vi "Measurement Logic.vi"() -> ()   [LabVIEW 2021, in "Quiescent Current_Channel Ganging.lvlib"]
uses:
  Quiescent Current_Channel Ganging.lvlib
  <vilib>/Plug-In SDKs/Measurements/Measure Call Context/Measure Call Context.lvclass
  Measurement Configuration.ctl
  Measurement Results.ctl
  <instrlib>/niDCPower/nidcpower.llb/niDCPower Source Mode.ctl
  <instrlib>/niDCPower/nidcpower.llb/niDCPower Output Function.ctl
panel:
  out "measurement results":T1
  in  "measurement configuration":T2={"DUT setup time"=1.0, "Source delay"=0.005, "Aperture time"=0.005, "Source master resource name"="Lorem ipsum dolor sit", "Source slave resource names"=["", ""], "Source system configuration"=enum."Parallel", "Source start voltage"=1.0, "Source stop voltage"=1.0, "Source voltage sweep points"=1, "Source voltage level range"=32.0, "Source sense"=-64, "Source limit symmetry"=enum."Asymmetric", "Source current limit range"=64.0, "Source current limit low"=-32.0, "Source current limit high"=-32.0, "Source transient response"=-64, "Source voltage gain bandwidth"=1.0, "Source voltage compensation frequency"=3530.0, "Source voltage pole-zero ratio"=2.0} {"Source start voltage" format="%#_6p"; "Source sense" items=["Local"=1008, "Remote"=1009]; "Source transient response" items=["Slow"=1041, "Normal"=1038, "Fast"=1039, "Custom"=1042]; "Source voltage level range" format="%#_6p"}
  out "measure call context out":refnum<class "Measure Call Context.lvclass">
  in  "measure call context in":refnum<class "Measure Call Context.lvclass">
  out "error out":errorcluster
  in  "error in":errorcluster
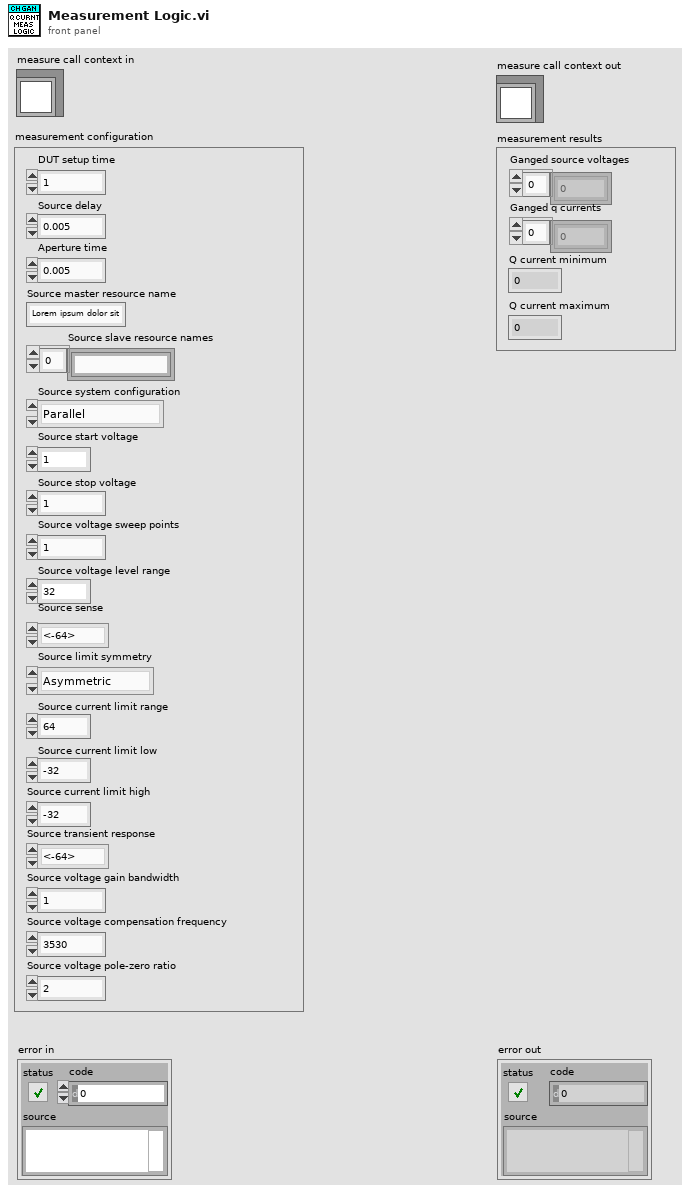
[diagram p1: front panel]
types:
  T1 = typedef "Quiescent Current_Channel Ganging.lvlib/Measurement Results.ctl" = cluster{"Ganged source voltages":dbl[], "Ganged q currents":dbl[], "Q current minimum":dbl, "Q current maximum":dbl}
  T2 = typedef "Quiescent Current_Channel Ganging.lvlib/Measurement Configuration.ctl" = cluster{"DUT setup time":dbl, "Source delay":dbl, "Aperture time":dbl, "Source master resource name":string, "Source slave resource names":string[], "Source system configuration":enum32{"Series", "Parallel", "Manual"}, "Source start voltage":dbl, "Source stop voltage":dbl, "Source voltage sweep points":i32, "Source voltage level range":dbl, "Source sense":i32, "Source limit symmetry":enum32{"Symmetric", "Asymmetric"}, "Source current limit range":dbl, "Source current limit low":dbl, "Source current limit high":dbl, "Source transient response":i32, "Source voltage gain bandwidth":dbl, "Source voltage compensation frequency":dbl, "Source voltage pole-zero ratio":dbl}
  T3 = typedef "niDCPower Output Function.ctl" = i32
  T4 = typedef "niDCPower Source Mode.ctl" = i32
  T5 = typedef "NIDCPower_channel_ganging - ctl - channel def.ctl" = cluster{"resource name":refnum<k15>, "channels":string, "Channel Mode":T6}
  T6 = typedef "NIDCPower_channel_ganging - ctl - channel mode.ctl" = enum32{"Master", "Slave", "Slave - Inverted"}
  T7 = typedef "NIDCPower_channel_ganging - ctl - ganged session.ctl" = cluster{"Ganged Config":T8, "Session List":refnum<k15>[], "Session Mode":T6[], "Channel":string[]}
  T8 = typedef "NIDCPower_channel_ganging - ctl - ganged config.ctl" = enum32{"Series", "Parallel", "Manual"}
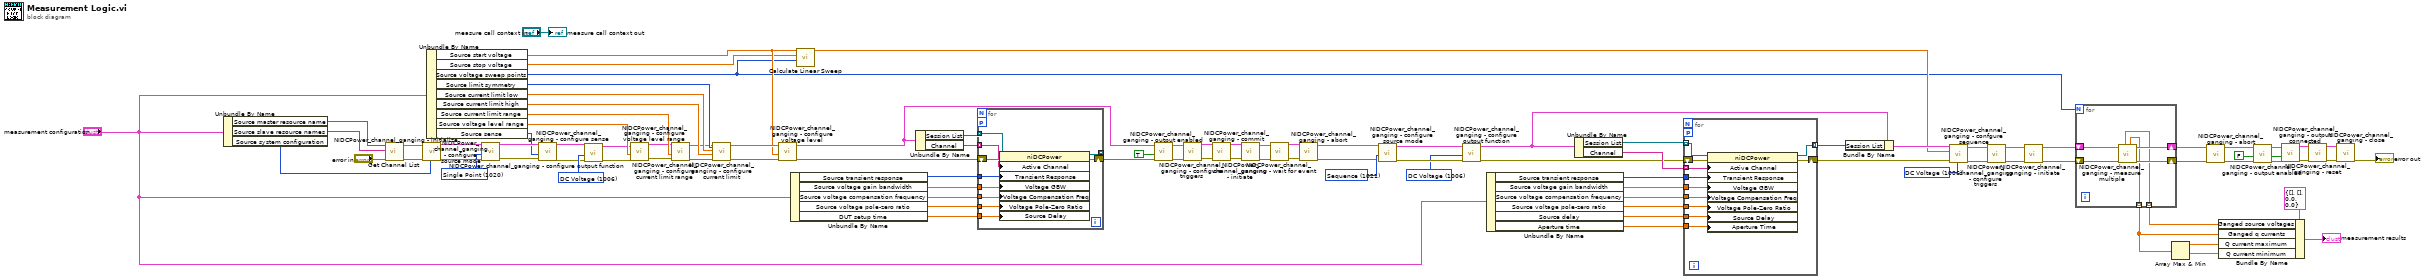
[diagram p0: block diagram]
diagram:
  w30 = T3 1006 items=["DC Voltage"=1006, "DC Current"=1007, "Pulse Voltage"=1049, "Pulse Current"=1050] ("output function")
  w37 = T3 1006 items=["DC Voltage"=1006, "DC Current"=1007, "Pulse Voltage"=1049, "Pulse Current"=1050] ("output function")
  w39 = T4 1021 items=["Single Point"=1020, "Sequence"=1021] ("source mode")
  w44 = FALSE ("output enabled")
  w88 = T3 1006 items=["DC Voltage"=1006, "DC Current"=1007, "Pulse Voltage"=1049, "Pulse Current"=1050] ("output function")
  w96 = T4 1020 items=["Single Point"=1020, "Sequence"=1021] ("source mode")
  n1 = Unbundle By Name("measurement configuration") -> ("Source master resource name"=w57:string, "Source slave resource names"=w56:string[], "Source system configuration"=w89:enum32{"Series", "Parallel", "Manual"})
  n2 = call "Get Channel List.vi"("error in (no error)"="error in", "Slave resource names"=w56, "Master resouce name"=w57) -> ("error out"=w58:errorcluster, "Channel List"=w59:T5[])  [unwired: 7 in]
  n3 = call "NIDCPower_channel_ganging - initialize.vi"("Ganged Config"=w89, "error in (no error)"=w58, "Channel List"=w59) -> ("error out"=w97:errorcluster, "Ganged Session Out"=w98:T7)  [unwired: 7 in]
  n4 = Unbundle By Name("measurement configuration") -> ("Source start voltage"=w49:dbl, "Source stop voltage"=w48:dbl, "Source voltage sweep points"=w8:i32, "Source limit symmetry"=w90:enum32{"Symmetric", "Asymmetric"}, "Source current limit low"=w91:dbl, "Source current limit high"=w92:dbl, "Source current limit range"=w93:dbl, "Source voltage level range"=w94:dbl, "Source sense"=w60:i32)
  n5 = call "NIDCPower_channel_ganging - configure source mode.vi"("error in (no error)"=w97, "source mode"=w96, "Ganged Session In"=w98) -> ("error out"=w80:errorcluster, "Ganged Session Out"=w81:T7)  [unwired: 7 in]
  n6 = call "NIDCPower_channel_ganging - configure sense.vi"("error in (no error)"=w80, "sense"=w60, "Ganged Session In"=w81) -> ("error out"=w78:errorcluster, "Ganged Session Out"=w79:T7)  [unwired: 7 in]
  n7 = call "NIDCPower_channel_ganging - configure output function.vi"("error in (no error)"=w78, "output function"=w88, "Ganged Session In"=w79) -> ("error out"=w76:errorcluster, "Ganged Session Out"=w77:T7)  [unwired: 7 in]
  n8 = call "NIDCPower_channel_ganging - configure voltage level range.vi"("error in (no error)"=w76, "voltage level range"=w94, "Ganged Session In"=w77) -> ("error out"=w84:errorcluster, "Ganged Session Out"=w87:T7)  [unwired: 7 in]
  n9 = call "NIDCPower_channel_ganging - configure current limit range.vi"("error in (no error)"=w84, "current limit range"=w93, "Ganged Session In"=w87) -> ("error out"=w83:errorcluster, "Ganged Session Out"=w86:T7)  [unwired: 7 in]
  n10 = call "NIDCPower_channel_ganging - configure current limit.vi"("Limit Symmetry"=w90, "error in (no error)"=w83, "Current limit/hi"=w92, "Current limit lo"=w91, "Ganged Session In"=w86) -> ("error out"=w82:errorcluster, "Ganged Session Out"=w85:T7)  [unwired: 5 in]
  n11 = call "NIDCPower_channel_ganging - configure voltage level.vi"("error in (no error)"=w82, "voltage level"=w49, "Ganged Session In"=w85) -> ("error out"=w65:errorcluster, "Ganged Session Out"=w61:T7)  [unwired: 7 in]
  n12 = Unbundle By Name("measurement configuration") -> ("Source transient response"=w55:i32, "Source voltage gain bandwidth"=w53:dbl, "Source voltage compensation frequency"=w52:dbl, "Source voltage pole-zero ratio"=w51:dbl, "DUT setup time"=w54:dbl)
  n13 = call "Calculate Linear Sweep.vi"("Points"=w8, "Stop level"=w48, "Start level"=w49) -> ("Values"=w14:dbl[])  [unwired: 8 in]
  n14 = Unbundle By Name(w61) -> ("Session List"=w63:refnum<k15>[], "Channel"=w62:string[])
  n15 = for {
    tunnel: [w109] -> _ mode=indexing
    shift-right: [w107] -> w64
    shift-left: w65 -> [w108]
    workers-P: _ -> [_]
    tunnel: w63 -> [w106] mode=indexing
    tunnel: w62 -> [w105] mode=indexing
    tunnel: w55 -> [w104]
    tunnel: w54 -> [w103]
    tunnel: w53 -> [w102]
    tunnel: w52 -> [w101]
    tunnel: w51 -> [w100]
    n16 = property class="niDCPower"(reference=w106, error in=w108, "Active Channel"=w105, "Transient Response"=w104, "Voltage GBW"=w102, "Voltage Compensation Freq"=w101, "Voltage Pole-Zero Ratio"=w100, "Source Delay"=w103) -> (reference out=w109:refnum<k15>, error out=w107:errorcluster)
  }
  n17 = call "NIDCPower_channel_ganging - output enabled.vi"("error in (no error)"=w64, "output enabled"=TRUE, "Ganged Session In"=w61) -> ("error out"=w68:errorcluster, "Ganged Session Out"=w69:T7)  [unwired: 7 in]
  n18 = call "NIDCPower_channel_ganging - configure triggers.vi"("error in (no error)"=w68, "Ganged Session In"=w69) -> ("error out"=w66:errorcluster, "Ganged Session Out"=w67:T7)  [unwired: 8 in]
  n19 = call "NIDCPower_channel_ganging - commit.vi"("error in (no error)"=w66, "Ganged Session In"=w67) -> ("error out"=w71:errorcluster, "Ganged Session Out"=w70:T7)  [unwired: 8 in]
  n20 = call "NIDCPower_channel_ganging - initiate.vi"("error in (no error)"=w71, "Ganged Session In"=w70) -> ("error out"=w73:errorcluster, "Ganged Session Out"=w72:T7)  [unwired: 8 in]
  n21 = call "NIDCPower_channel_ganging - wait for event.vi"("error in (no error)"=w73, "Ganged Session in"=w72) -> ("error out"=w75:errorcluster, "Ganged Session Out"=w74:T7)  [unwired: 8 in]
  n22 = call "NIDCPower_channel_ganging - abort.vi"("error in (no error)"=w75, "Ganged Session In"=w74) -> ("error out"=w29:errorcluster, "Ganged Session Out"=w28:T7)  [unwired: 8 in]
  n23 = call "NIDCPower_channel_ganging - configure source mode.vi"("error in (no error)"=w29, "source mode"=w39, "Ganged Session In"=w28) -> ("error out"=w40:errorcluster, "Ganged Session Out"=w41:T7)  [unwired: 7 in]
  n24 = call "NIDCPower_channel_ganging - configure output function.vi"("error in (no error)"=w40, "output function"=w37, "Ganged Session In"=w41) -> ("error out"=w23:errorcluster, "Ganged Session Out"=w38:T7)  [unwired: 7 in]
  n25 = Unbundle By Name("measurement configuration") -> ("Source transient response"=w24:i32, "Source voltage gain bandwidth"=w22:dbl, "Source voltage compensation frequency"=w21:dbl, "Source voltage pole-zero ratio"=w20:dbl, "Source delay"=w19:dbl, "Aperture time"=w18:dbl)
  n26 = Unbundle By Name(w38) -> ("Session List"=w26:refnum<k15>[], "Channel"=w25:string[])
  n27 = for {
    tunnel: w26 -> [w120] mode=indexing
    tunnel: w25 -> [w112] mode=indexing
    tunnel: w24 -> [w119]
    workers-P: _ -> [_]
    tunnel: w22 -> [w117]
    tunnel: w21 -> [w116]
    tunnel: w20 -> [w115]
    tunnel: w19 -> [w114]
    tunnel: w18 -> [w113]
    shift-right: [w111] -> w16
    shift-left: w23 -> [w118]
    tunnel: [w110] -> w17 mode=indexing
    n28 = property class="niDCPower"(reference=w120, error in=w118, "Active Channel"=w112, "Transient Response"=w119, "Voltage GBW"=w117, "Voltage Compensation Freq"=w116, "Voltage Pole-Zero Ratio"=w115, "Source Delay"=w114, "Aperture Time"=w113) -> (reference out=w110:refnum<k15>, error out=w111:errorcluster)
  }
  n29 = Bundle By Name(cluster=w38, "Session List"=w17) -> (w32:T7)
  n30 = call "NIDCPower_channel_ganging - confgure sequence.vi"("output function"=w30, "error in (no error)"=w16, "Values"=w14, "Ganged Session In"=w32) -> ("error out"=w31:errorcluster, "Ganged Session Out"=w15:T7)  [unwired: 6 in]
  n31 = call "NIDCPower_channel_ganging - configure triggers.vi"("error in (no error)"=w31, "Ganged Session In"=w15) -> ("error out"=w42:errorcluster, "Ganged Session Out"=w43:T7)  [unwired: 8 in]
  n32 = call "NIDCPower_channel_ganging - initiate.vi"("error in (no error)"=w42, "Ganged Session In"=w43) -> ("error out"=w11:errorcluster, "Ganged Session Out"=w13:T7)  [unwired: 8 in]
  n33 = for {
    N: w8 -> [_]
    shift-right: [w123] -> w10
    shift-left: w11 -> [w126]
    shift-right: [w124] -> w12
    shift-left: w13 -> [w125]
    tunnel: [w122] -> w2 mode=indexing
    tunnel: [w121] -> w1 mode=indexing
    n34 = call "NIDCPower_channel_ganging - measure multiple.vi"("error in (no error)"=w126, "Ganged Session In"=w125) -> ("error out"=w123:errorcluster, "Ganged Session Out"=w124:T7, "ganged current measurement"=w121:dbl, "ganged voltage measurement"=w122:dbl)  [unwired: 2 in, 4 out]
  }
  n35 = Array Max & Min(array=w1) -> (max value=w4:dbl, min value=w3:dbl)  [unwired: 2 out]
  n36 = call "NIDCPower_channel_ganging - abort.vi"("error in (no error)"=w10, "Ganged Session In"=w12) -> ("error out"=w9:errorcluster, "Ganged Session Out"=w45:T7)  [unwired: 8 in]
  n37 = Bundle By Name(cluster=T1 {"Ganged source voltages"=[], "Ganged q currents"=[], "Q current minimum"=0.0, "Q current maximum"=0.0} ("Measurement Results"), "Ganged source voltages"=w2, "Ganged q currents"=w1, "Q current maximum"=w4, "Q current minimum"=w3) -> (→"measurement results":T1)
  n38 = call "NIDCPower_channel_ganging - output enabled.vi"("error in (no error)"=w9, "output enabled"=w44, "Ganged Session In"=w45) -> ("error out"=w47:errorcluster, "Ganged Session Out"=w46:T7)  [unwired: 7 in]
  n39 = call "NIDCPower_channel_ganging - output connected.vi"("error in (no error)"=w47, "output enabled"=w44, "Ganged Session In"=w46) -> ("error out"=w35:errorcluster, "Ganged Session Out"=w36:T7)  [unwired: 7 in]
  n40 = call "NIDCPower_channel_ganging - reset.vi"("error in (no error)"=w35, "Ganged Session In"=w36) -> ("error out"=w33:errorcluster, "Ganged Session Out"=w34:T7)  [unwired: 8 in]
  n41 = call "NIDCPower_channel_ganging - close.vi"("error in (no error)"=w33, "Ganged Session In"=w34) -> ("error out"=→"error out":errorcluster)  [unwired: 9 in]
  "measure call context out" <- "measure call context in"
